vi "test2021.vi"() -> ()   [LabVIEW 2020]
panel:
  out "Boolean 2":bool
  out "Boolean":bool
  out "result":dbl
  out "Numeric 5":u8
  out "Numeric 4":u8
  out "output":i32
  out "Numeric 3":u8
  in  "Numeric 2":u8
  in  "Numeric":u8
  out "sum":dbl
  out "XY Graph":cluster{dbl[], dbl[]}[](graph)
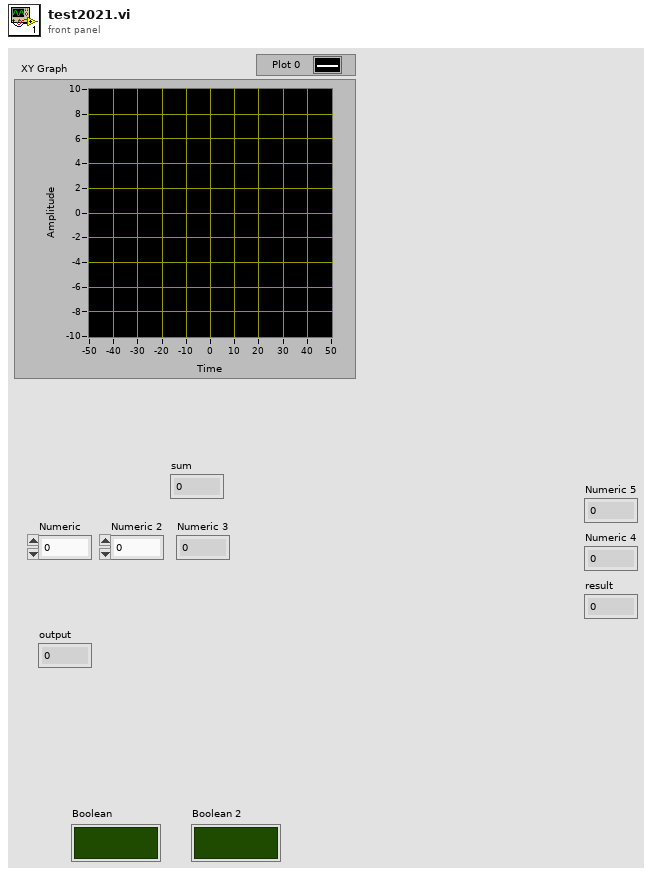
[diagram p1: front panel]
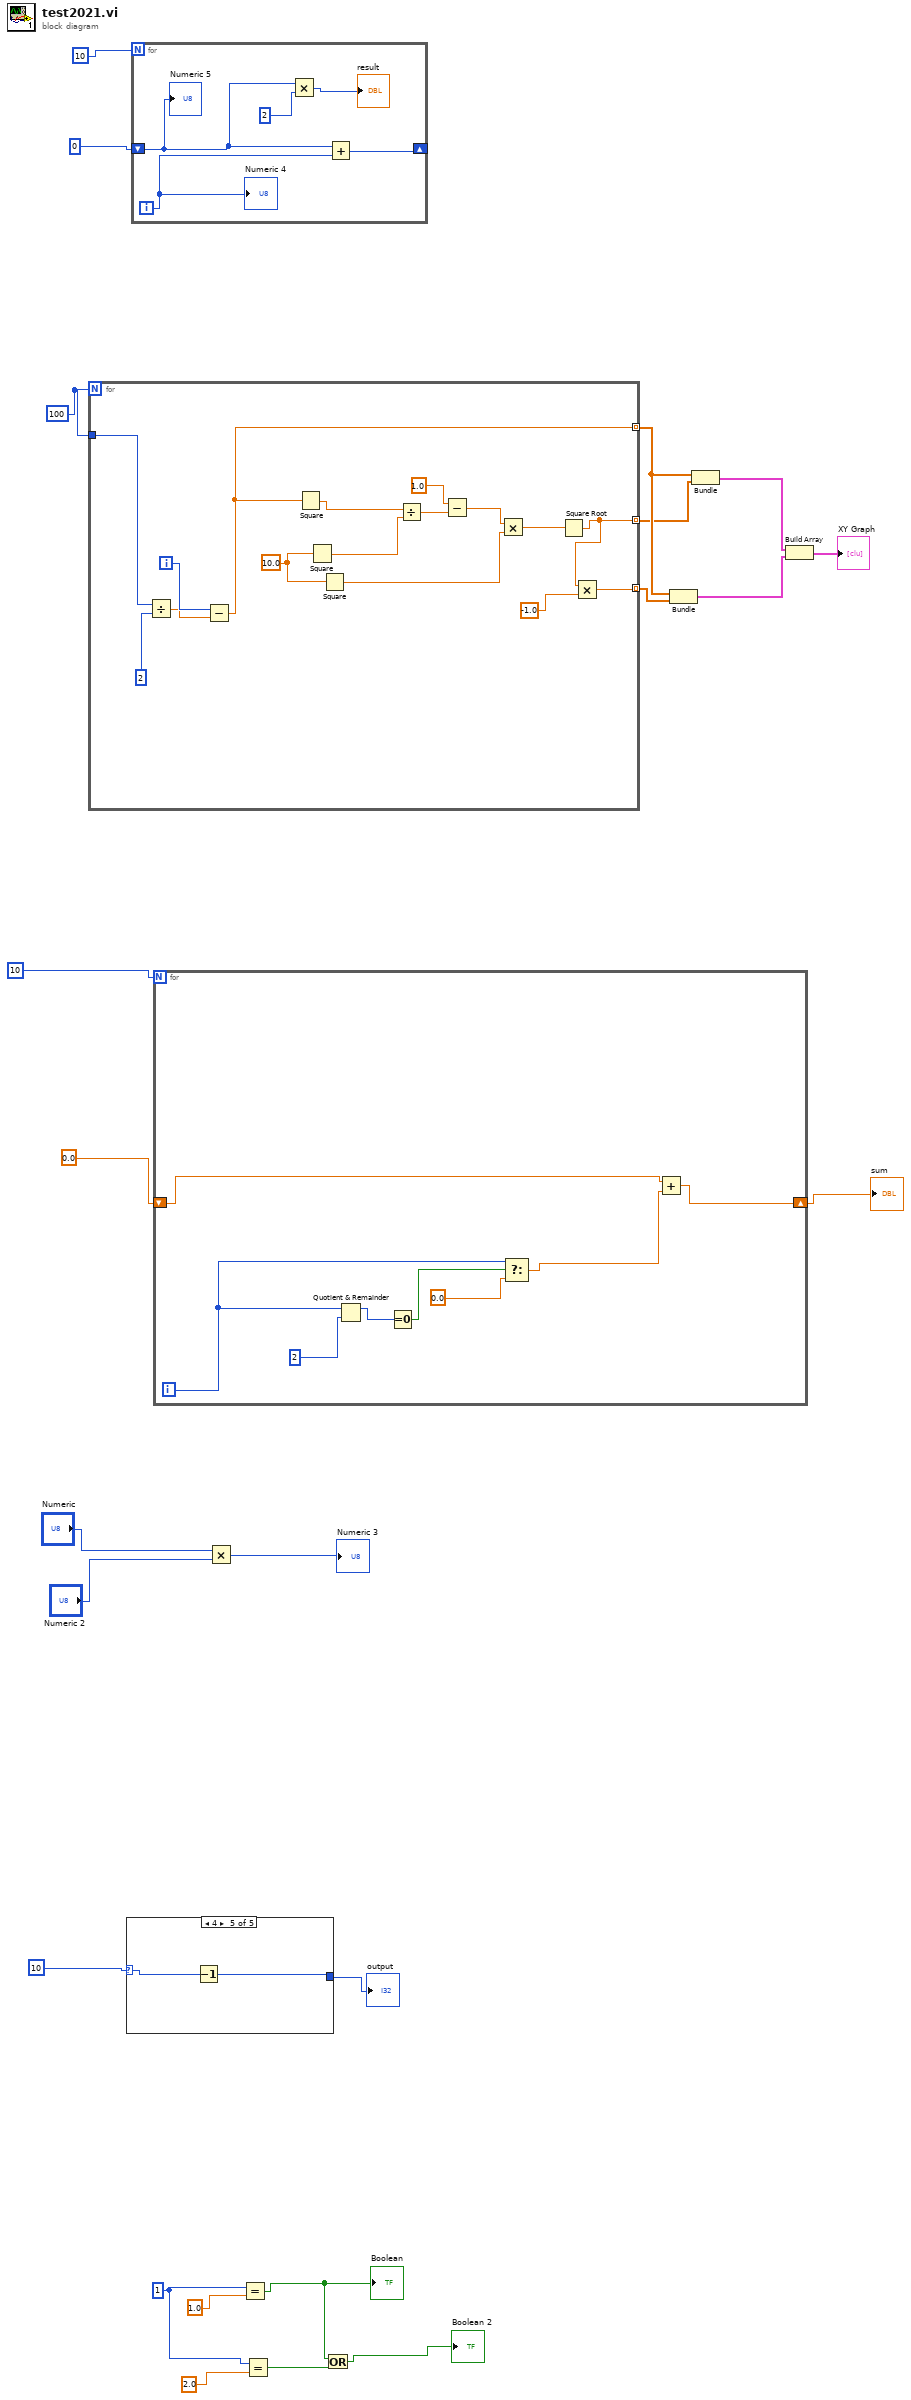
[diagram p0: block diagram]
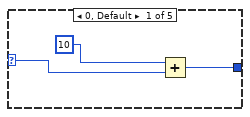
[diagram p2: hidden frame]
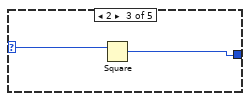
[diagram p4: hidden frame]
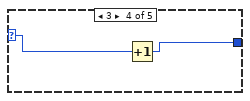
[diagram p5: hidden frame]
diagram:
  w6 = 1
  w23 = 100
  n1 = for {
    N: w23 -> [_]
    tunnel: w23 -> [w39]
    tunnel: [w35] -> w21 mode=indexing
    tunnel: [w25] -> w20 mode=indexing
    tunnel: [w24] -> w22 mode=indexing
    i -> [w37]
    w34 = 10.0
    n2 = Divide(x=w39, y=2) -> (x/y=w36:dbl)
    n3 = Subtract(x=w37, y=w36) -> (x-y=w35:dbl)
    n4 = Square(x=w35) -> (x^2=w33:dbl)
    n5 = Square(x=w34) -> (x^2=w32:dbl)
    n6 = Square(x=w34) -> (x^2=w28:dbl)
    n7 = Divide(x=w33, y=w32) -> (x/y=w31:dbl)
    n8 = Subtract(x=1.0, y=w31) -> (x-y=w29:dbl)
    n9 = Multiply(x=w29, y=w28) -> (x*y=w27:dbl)
    n10 = Square Root(x=w27) -> (sqrt(x)=w25:dbl)
    n11 = Multiply(x=w25, y=-1.0) -> (x*y=w24:dbl)
  }
  n12 = case shown="4" 10 {
    selector: 10 -> [w41 w43 w45 w47 w49]
    tunnel: [w40 w43 w44 w46 w48] -> w9
    frame 0, Default {
      n13 = Add(x=10, y=w41) -> (x+y=w40:i32)
    }
    frame 1 {
    }
    frame 2 {
      n14 = Square(x=w45) -> (x^2=w44:i32)
    }
    frame 3 {
      n15 = Increment(x=w47) -> (x+1=w46:i32)
    }
    frame 4 {
      n16 = Decrement(x=w49) -> (x-1=w48:i32)
    }
  }
  "output" <- w9
  n17 = for {
    N: 10 -> [_]
    shift-right: [w50] -> _
    shift-left: 0 -> [w52]
    i -> [w51]
    n18 = Multiply(x=w52, y=2) -> (x*y=→"result":i32)
    n19 = Add(x=w52, y=w51) -> (x+y=w50:i32)
    "Numeric 5" <- w52
    "Numeric 4" <- w51
  }
  n20 = for {
    N: 10 -> [_]
    shift-right: [w55] -> w14
    shift-left: 0.0 -> [w62]
    i -> [w58]
    n21 = Quotient & Remainder(x=w58, y=2) -> (x-y*floor(x/y)=w60:i32)  [unwired: 1 out]
    n22 = Equal To 0?(x=w60) -> (x = 0?=w59:bool)
    n23 = Select(t=w58, s=w59, f=0.0) -> (s? t:f=w56:dbl)
    n24 = Add(x=w62, y=w56) -> (x+y=w55:dbl)
  }
  "sum" <- w14
  n25 = Multiply(x="Numeric", y="Numeric 2") -> (x*y=→"Numeric 3":u8)
  n26 = Equal?(x=w6, y=1.0) -> (x = y?=w2:bool)
  "Boolean" <- w2
  n27 = Equal?(x=w6, y=2.0) -> (x = y?=w3:bool)
  n28 = Or(x=w2, y=w3) -> (x .or. y?=→"Boolean 2":bool)
  n29 = Bundle(w21, w22) -> (w18:cluster{dbl[], dbl[]})  [unwired: 1 in]
  n30 = Bundle(w21, w20) -> (w19:cluster{dbl[], dbl[]})  [unwired: 1 in]
  n31 = Build Array(w19, w18) -> (→"XY Graph":cluster{dbl[], dbl[]}[])
